vi "SGL_K2_xdelay_dot.vi"(8 "ND":u16=9, 10 "X":sgl[](array[numeric])=[1.0, 2.0, 3.0, 4.0, 5.0, 6.0, 7.0, 8.0, 9.0, 0.0, 0.0, 0.0, 0.0, 0.0, 0.0, 0.0, 0.0, 0.0, 0.0, 0.0, 0.0, 0.0, 0.0, 0.0], 11 "Refnum in":refnum<k21>="K2") -> (2 "Numeric":sgl format="%#_13g")   [LabVIEW 2017]
doc: "Given an input array X and a reference to a memory item, comput the dot product,\neg K.*X. X can be a vector up to length = 24.\n\nND is the size of the vectors.\n\n\nTHIS VI IS DIFFERENT FROM \"SGL Row matrix multiply loop\" by different sizes allowed."
uses:
  <vilib>/Platform/TimedLoop/XDataNode/timing_clust.ctl
  <vilib>/Platform/TimedLoop/XDataNode/nitl_modes.ctl
  <vilib>/Platform/TimedLoop/XDataNode/wakeup.ctl
  <vilib>/rvi/Emulation/niFpgaSctlEmulationGetInTimedLoop.vi
  <vilib>/rvi/Emulation/niFpgaEmulationReportErrorSimple.vi
  <vilib>/rvi/Emulation/niFpgaGetClockAttributes.vi
  <vilib>/rvi/Emulation/niFpgaCriticalErrorInLSC.vi
  <vilib>/rvi/DataTransferAndStorage/Container/Common/niFpgaContainerExecOnDevCompGetState.vi
  <vilib>/rvi/Emulation/niFpgaEmulationIsFPGAContextNoSignature.vi
  <vilib>/rvi/DataTransferAndStorage/Container/Common/niFpgaContainerGetUniqueNameForEmu.vi
  <vilib>/rvi/Emulation/niFpgaProcessEmulError.vi
  <vilib>/rvi/errors/nirviReportUnexpectedCaseInternalError (U32).vi
  <vilib>/rvi/Memory/Memory_Emulation/niFpgaMemoryEmulationCacheClearOnFirstRun.vi
  <vilib>/rvi/Memory/Memory_Emulation/nirvimemoryEmulationManagerCache_MakeExclusive.vi
  <vilib>/rvi/Memory/Memory_Emulation/niFpgaMemoryEmulationValidateCache.vi
  <vilib>/rvi/Memory/Memory_Emulation/nirvimemoryEmulationManagerCache_InsertValue.vi
  <vilib>/Utility/error.llb/Clear Errors.vi
  <vilib>/rvi/Memory/Memory_Emulation/nirvimemoryEmulationManagerCache_ReleaseExclusive.vi
  <vilib>/rvi/Memory/Memory_Emulation/nirvimemoryEmulationManagerCache_GetValue.vi
  <vilib>/rvi/Memory/Memory_Emulation/nirvimemoryEmulationManagerCache_SetValue.vi
  <vilib>/rvi/Emulation/niFpgaSctlEmulationResourceMgr.vi
  <vilib>/Platform/TimedLoop/XDataNode/XDataNode.xnode
  <vilib>/rvi/DataTransferAndStorage/Container/XNode/niFpgaContainer.xnode
  <vilib>/rvi/Memory/Memory_Emulation/niFpgaMemoryEmulationRefIn.vi
  <vilib>/Platform/TimedLoop/XDataNode/XDNodeRunTimeDep.lvlib
panel:
  # "The only difference between this and the other dot product \nis the size of the array we accept. This is good for ND=24. But I don't want to take\nup all that room in the other one since there are many instances."
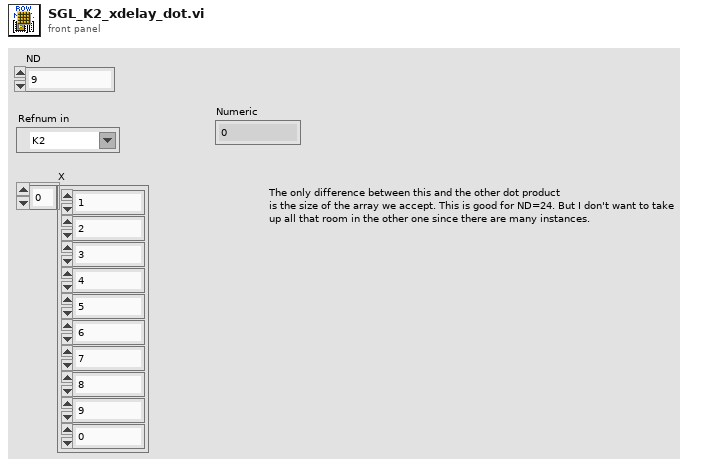
[diagram p1: front panel]
types:
  T1 = typedef "XDNodeRunTimeDep.lvlib/timing_clust.ctl" = cluster{"Expected End [f-1]":u64, "Actual End [f-1]":u64, "Finished Late? [f-1]":bool, "Expected End [i-1]":u64, "Actual End [i-1]":u64, "Finished Late? [i-1]":bool, "Expected Start [i]":u64, "Actual Start [i]":u64, "Expected Start [f]":u64, "Actual Start [f]":u64, "Source Name":string, "Structure Name":string, "Period":i64, "Deadline":i64, "Offset":i64, "Start":i64, "Priority":i32, "Timeout":i32, "Mode":T2, "Wakeup Reason":T3, "Error":errorcluster, "Source Type":string, "Secondary Source Type":string, "Global End Time":u64, "Global Start Time":u64, "Frame Duration":u64, "Iteration Duration":u64, "Assigned CPU":i32, "I/O Scan Engine Mode":u32}
  T2 = typedef "XDNodeRunTimeDep.lvlib/nitl_modes.ctl" = enum32{"No Change", "Process missed periods, maintain original phase", "Discard missed periods, maintain original phase", "Process missed periods, ignore original phase", "Discard missed periods, ignore original phase"}
  T3 = typedef "XDNodeRunTimeDep.lvlib/wakeup.ctl" = enum32{"Normal", "Aborted", "Asynchronous wakeup", "Timing source error", "Timed loop error", "Timeout"}
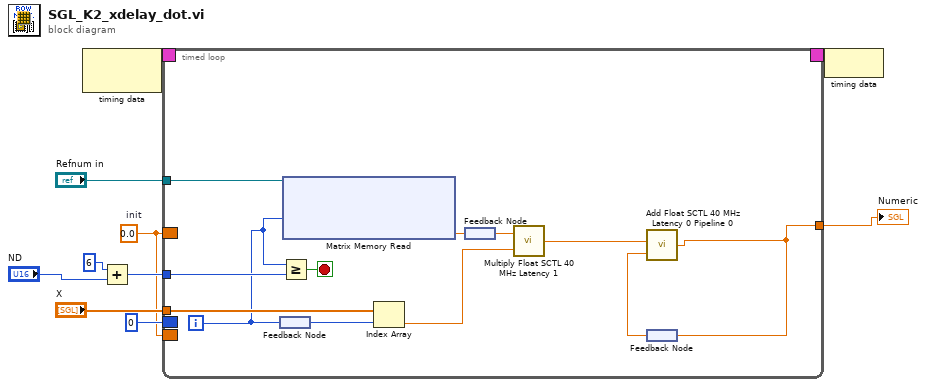
[diagram p0: block diagram]
diagram:
  w1 = sgl 0.0  # init
  n1 = node-c288() -> (w10:T1)  [unwired: 1 in]
  n2 = Add(x=6, y="ND") -> (x+y=w2:i32)
  n3 = timed-loop {
    timing: w10 -> [_]
    timing-out: [_] -> w9
    border: w1 -> [_]
    tunnel: "Refnum in" -> [w21]
    tunnel: "X" -> [w20]
    tunnel: [w16] -> w6
    border: 0 -> [_]
    tunnel: w2 -> [w18]
    border: w1 -> [_]
    i -> [w15]
    stop <- w22 stop-if-true
    n4 = feedback #1() -> (w19:i32)
    n5 = feedback-in #1(w15) -> ()
    n6 = Greater Or Equal?(x=w15, y=w18) -> (x >= y?=w22:bool)
    n7 = xnode "Matrix Memory Read"("Address"=w15, "Memory In"=w21) -> ("Data"=w11:sgl)  [unwired: 1 out]
    n8 = Index Array(array=w20, index=w19) -> (element=w13:sgl)
    n9 = feedback #2() -> (w12:sgl)
    n10 = feedback-in #2(w11) -> ()
    n11 = call "Multiply Float SCTL 40 MHz Latency 1.vi"("y"=w13, "x"=w12) -> ("x[k-1]*y[k-1]"=w14:sgl)
    n12 = feedback #3() -> (w17:sgl)
    n13 = call "Add Float SCTL 40 MHz Latency 0 Pipeline 0.vi"("y"=w17, "x"=w14) -> ("x+y"=w16:sgl)
    n14 = feedback-in #3(w16) -> ()
  }
  "Numeric" <- w6
  n15 = node-c288(w9) -> ()
